vi "Set Graticule.vi"(8 "error in (no error)":errorcluster, 11 "reference":refnum<vi>) -> (0 "error out":errorcluster)   [LabVIEW 2017]
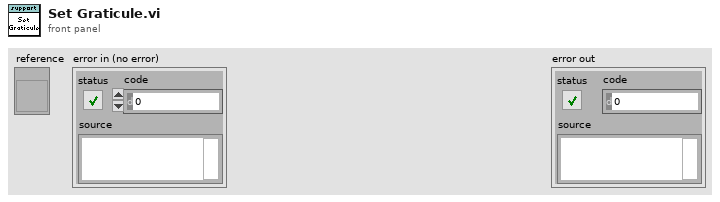
[diagram p1: front panel]
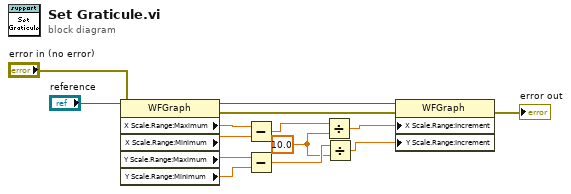
[diagram p0: block diagram]
diagram:
  w3 = 10.0 ("y")
  n1 = property on="Property Node" class="WFGraph"(reference="reference", error in="error in (no error)") -> (reference out=w4:refnum<vi>, error out=w6:errorcluster, "X Scale.Range:Maximum"=w12:dbl, "X Scale.Range:Minimum"=w11:dbl, "Y Scale.Range:Maximum"=w10:dbl, "Y Scale.Range:Minimum"=w9:dbl)
  n2 = Subtract(x=w12, y=w11) -> (x-y=w13:dbl)
  n3 = Subtract(x=w10, y=w9) -> (x-y=w14:dbl)
  n4 = Divide(x=w13, y=w3) -> (x/y=w7:dbl)
  n5 = Divide(x=w14, y=w3) -> (x/y=w8:dbl)
  n6 = property on="Property Node" class="WFGraph"(reference=w4, error in=w6, "X Scale.Range:Increment"=w7, "Y Scale.Range:Increment"=w8) -> (error out=→"error out":errorcluster)  [unwired: 1 out]
